vi "Activity Light - Pulse.vi"(7 "Name":string="Activity Light", 8 "error in (no error)":errorcluster, 9 "OFF Color":u32(colorbox), 10 "ON Color":u32(colorbox), 11 "Type":T1=enum."Active (Yellow)") -> (0 "error out":errorcluster)   [LabVIEW 2024, in "EQMF.lvlib" / "Status Utils.lvlib"]
uses:
  Status Utils.lvlib
  _Private/Activity Light Color Types.ctl
  _Private/Activity Light Q Item.ctl
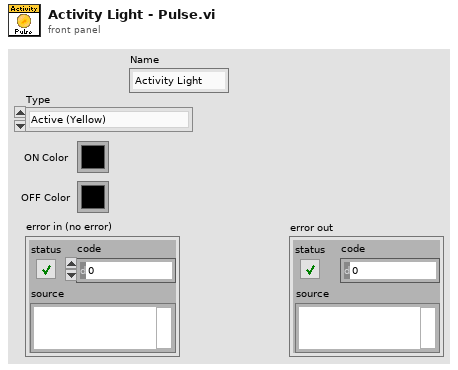
[diagram p1: front panel]
types:
  T1 = typedef "EQMF.lvlib/Status Utils.lvlib/Activity Light Color Types.ctl" = enum16{"OK (Green)", "Active (Yellow)", "Warning (Orange)", "Error (Red)", "Attention (Blue)", "Custom Color"}
  T2 = typedef "EQMF.lvlib/Status Utils.lvlib/Activity Light Q Item.ctl" = cluster{"Cmd":string, "Data":variant}
  T3 = cluster{"Type":T1, "ON Color":u32, "OFF Color":u32}
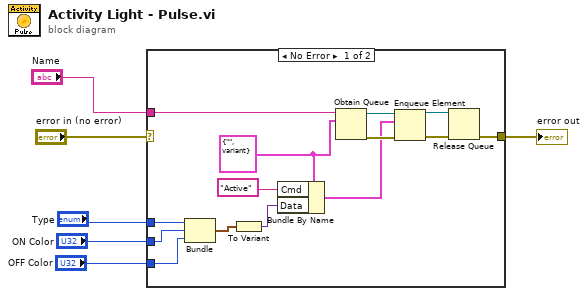
[diagram p0: block diagram]
diagram:
  n1 = case shown="No Error" "error in (no error)" {
    selector: "error in (no error)" -> [_ w21]
    tunnel: [w16 w21] -> w6
    tunnel: "Type" -> [w15 _]
    tunnel: "ON Color" -> [w14 _]
    tunnel: "OFF Color" -> [w8 _]
    tunnel: "Name" -> [w7 _]
    frame No Error {
      w11 = T2 {"Cmd"="", "Data"=variant} ("output cluster")
      n2 = Bundle("Type"=w15, "ON Color"=w14, "OFF Color"=w8) -> (w13:T3)  [unwired: 1 in]
      n3 = To Variant(anything=w13) -> (Variant=w10:variant)
      n4 = Bundle By Name(cluster=w11, "Cmd"="Active", "Data"=w10) -> (w9:T2)
      n5 = Obtain Queue(name (unnamed)=w7, element data type=w11) -> (queue out=w20:refnum<queue>, error out=w19:errorcluster)  [unwired: 3 in, 1 out]
      n6 = Enqueue Element(queue=w20, element=w9, error in (no error)=w19) -> (queue out=w17:refnum<queue>, error out=w18:errorcluster)  [unwired: 1 in, 1 out]
      n7 = Release Queue(queue=w17, error in (no error)=w18) -> (error out=w16:errorcluster)  [unwired: 1 in, 2 out]
    }
    frame Error {
    }
  }
  "error out" <- w6
